vi "START SALES.vi"(11 "REFERENCES":T1) -> ()   [LabVIEW 2019]
uses:
  Controls/References Cluster.ctl
  Controls/Custom Calendar/Custom Calendar.xctl
  <vilib>/Utility/miscctls.llb/LVRowAndColumnTypeDef.ctl
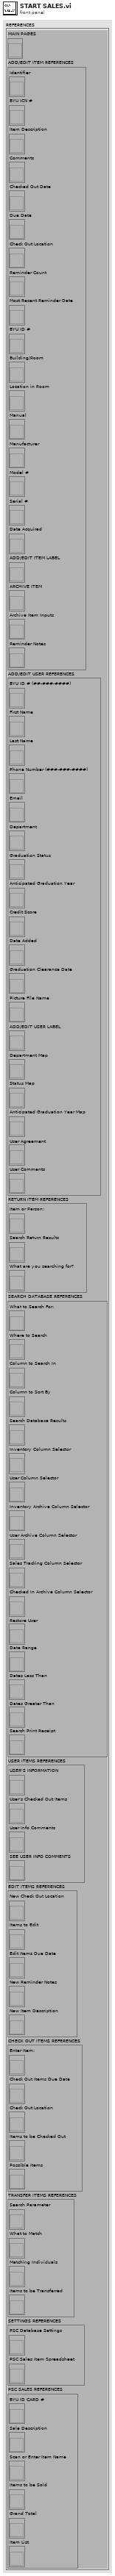
[diagram p1: front panel]
types:
  T1 = typedef "References Cluster.ctl" = cluster{"MAIN PAGES":refnum<vi>, "ADD/EDIT ITEM REFERENCES":cluster{"Identifier":refnum<vi>, "BYU ICN #":refnum<vi>, "Item Description":refnum<vi>, "Comments":refnum<vi>, "Checked Out Date":refnum<vi>, "Due Date":refnum<vi>, "Check Out Location":refnum<vi>, "Reminder Count":refnum<vi>, "Most Recent Reminder Date":refnum<vi>, "BYU ID #":refnum<vi>, "Building/Room":refnum<vi>, "Location in Room":refnum<vi>, "Manual":refnum<vi>, "Manufacturer":refnum<vi>, "Model #":refnum<vi>, "Serial #":refnum<vi>, "Date Acquired":refnum<vi>, "ADD/EDIT ITEM LABEL":refnum<vi>, "ARCHIVE ITEM":refnum<vi>, "Archive Item Inputs":refnum<vi>, "Reminder Notes":refnum<vi>}, "ADD/EDIT USER REFERENCES":cluster{"BYU ID # (##-###-####)":refnum<vi>, "First Name":refnum<vi>, "Last Name":refnum<vi>, "Phone Number (###-###-####)":refnum<vi>, "Email":refnum<vi>, "Department":refnum<vi>, "Graduation Status":refnum<vi>, "Anticipated Graduation Year":refnum<vi>, "Credit Score":refnum<vi>, "Date Added":refnum<vi>, "Graduation Clearance Date":refnum<vi>, "Picture File Name":refnum<vi>, "ADD/EDIT USER LABEL":refnum<vi>, "Department Map":refnum<vi>, "Status Map":refnum<vi>, "Anticipated Graduation Year Map":refnum<vi>, "User Agreement":refnum<vi>, "User Comments":refnum<vi>}, "RETURN ITEM REFERENCES":cluster{"Item or Person:":refnum<vi>, "Search Return Results":refnum<vi>, "What are you searching for?":refnum<vi>}, "SEARCH DATABASE REFERENCES":cluster{"What to Search For:":refnum<vi>, "Where to Search":refnum<vi>, "Column to Search In":refnum<vi>, "Column to Sort By":refnum<vi>, "Search Database Results":refnum<vi>, "Inventory Column Selector":refnum<vi>, "User Column Selector":refnum<vi>, "Inventory Archive Column Selector":refnum<vi>, "User Archive Column Selector":refnum<vi>, "Sales Tracking Column Selector":refnum<vi>, "Checked In Archive Column Selector":refnum<vi>, "Restore User":refnum<vi>, "Date Range":refnum<vi>, "Dates Less Than":refnum<vi>, "Dates Greater Than":refnum<vi>, "Search Print Receipt":refnum<vi>}, "USER ITEMS REFERENCES":cluster{"USER'S INFORMATION":refnum<vi>, "User's Checked Out Items":refnum<vi>, "User Info Comments":refnum<vi>, "SEE USER INFO COMMENTS":refnum<vi>}, "EDIT ITEMS REFERENCES":cluster{"New Check Out Location":refnum<vi>, "Items to Edit":refnum<vi>, "Edit Items Due Date":refnum<vi>, "New Reminder Notes":refnum<vi>, "New Item Description":refnum<vi>}, "CHECK OUT ITEMS REFERENCES":cluster{"Enter Item:":refnum<vi>, "Check Out Items Due Date":refnum<vi>, "Check Out Location":refnum<vi>, "Items to be Checked Out":refnum<vi>, "Possible Items":refnum<vi>}, "TRANSFER ITEMS REFERENCES":cluster{"Search Parameter":refnum<vi>, "What to Match":refnum<vi>, "Matching Individuals":refnum<vi>, "Items to be Transferred":refnum<vi>}, "SETTINGS REFERENCES":cluster{"PSC Database Settings":refnum<vi>, "PSC Sales Item Spreadsheet":refnum<vi>}, "PSC SALES REFERENCES":cluster{"BYU ID CARD #":refnum<vi>, "Sale Description":refnum<vi>, "Scan or Enter Item Name":refnum<vi>, "Items to be Sold":refnum<vi>, "Grand Total":refnum<vi>, "Item List":refnum<vi>}}
  T2 = typedef "LVRowAndColumnTypeDef.ctl" = cluster{"Row":i32, "Column":i32}
  T3 = cluster{"BYU ID CARD #":refnum<vi>, "Sale Description":refnum<vi>, "Scan or Enter Item Name":refnum<vi>, "Items to be Sold":refnum<vi>, "Grand Total":refnum<vi>, "Item List":refnum<vi>}
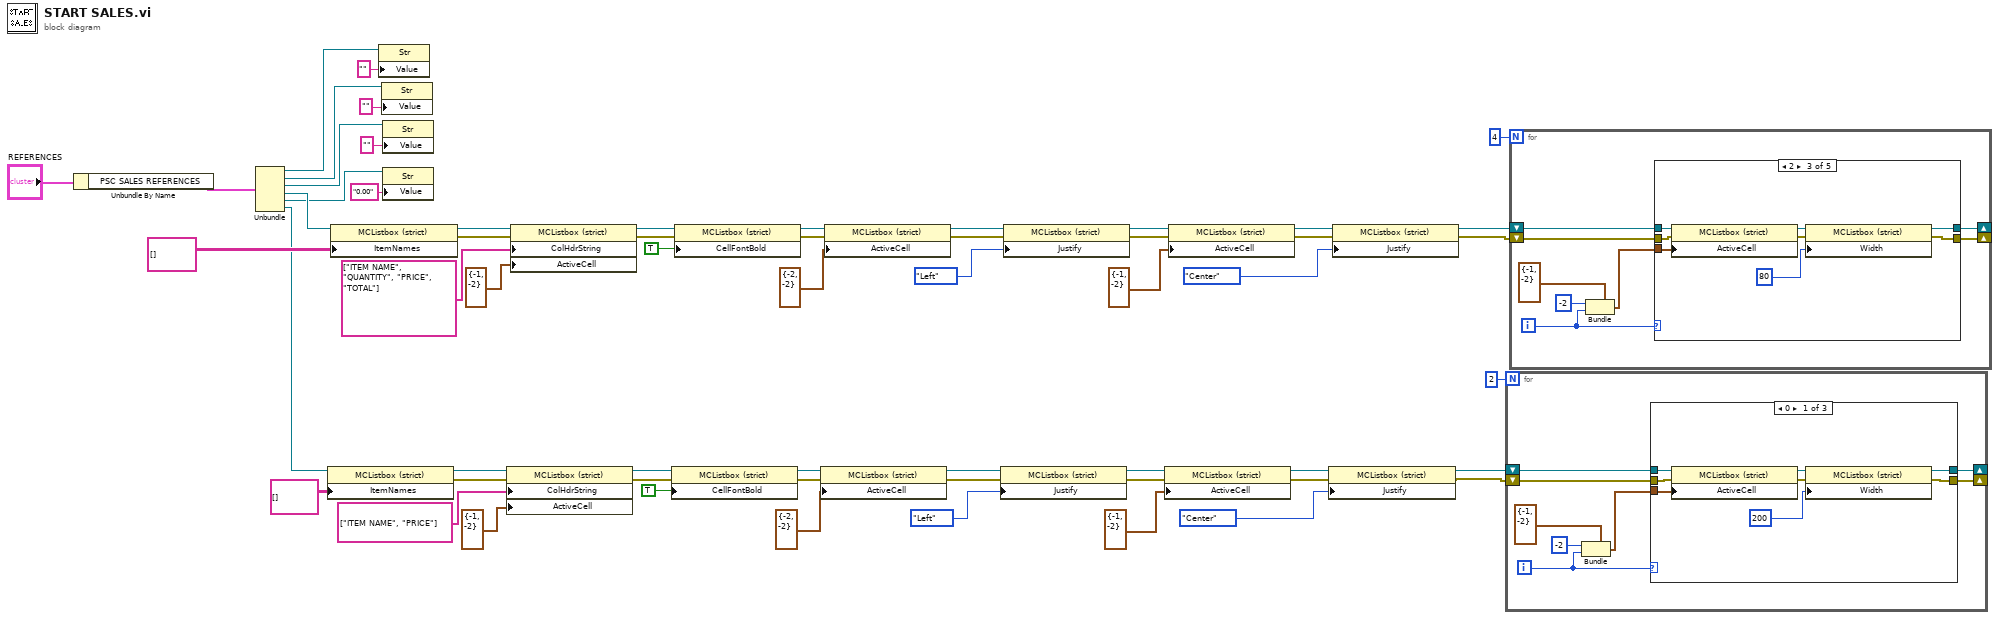
[diagram p0: block diagram]
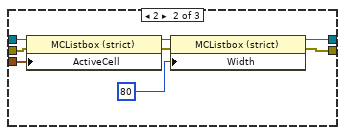
[diagram p2: hidden frame]
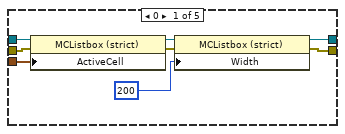
[diagram p4: hidden frame]
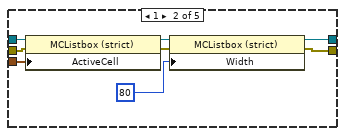
[diagram p5: hidden frame]
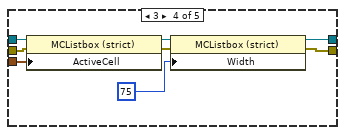
[diagram p6: hidden frame]
diagram:
  n1 = Unbundle By Name("REFERENCES") -> ("PSC SALES REFERENCES"=w57:T3)
  n2 = Unbundle(w57) -> ("BYU ID CARD #"=w32:refnum<vi>, "Sale Description"=w29:refnum<vi>, "Scan or Enter Item Name"=w27:refnum<vi>, "Items to be Sold"=w38:refnum<vi>, "Grand Total"=w25:refnum<vi>, "Item List"=w1:refnum<vi>)
  n3 = property class="MCListbox (strict)"(reference=w1, "ItemNames"=string[][] [] ("Item Names")) -> (reference out=w8:refnum<vi>, error out=w7:errorcluster)  [unwired: 1 in]
  n4 = property class="MCListbox (strict)"(reference=w38, "ItemNames"=string[][] [] ("Item Names")) -> (reference out=w40:refnum<vi>, error out=w39:errorcluster)  [unwired: 1 in]
  n5 = property class="Str"(reference=w32, "Value"="") -> ()  [unwired: 1 in, 2 out]
  n6 = property class="Str"(reference=w29, "Value"="") -> ()  [unwired: 1 in, 2 out]
  n7 = property class="Str"(reference=w27, "Value"="") -> ()  [unwired: 1 in, 2 out]
  n8 = property class="Str"(reference=w25, "Value"="0.00") -> ()  [unwired: 1 in, 2 out]
  n9 = property class="MCListbox (strict)"(reference=w8, error in=w7, "ColHdrString"=string[] ["ITEM NAME", "PRICE"] ("Column Header Strings[]"), "ActiveCell"=T2 {"Row"=-1, "Column"=-2} ("Active Cell:Active Cell")) -> (reference out=w23:refnum<vi>, error out=w22:errorcluster)
  n10 = property class="MCListbox (strict)"(reference=w40, error in=w39, "ColHdrString"=string[] ["ITEM NAME", "QUANTITY", "PRICE", "TOTAL"] ("Column Header Strings[]"), "ActiveCell"=T2 {"Row"=-1, "Column"=-2} ("Active Cell:Active Cell")) -> (reference out=w55:refnum<vi>, error out=w54:errorcluster)
  n11 = property class="MCListbox (strict)"(reference=w23, error in=w22, "CellFontBold"=TRUE ("Active Cell:Cell Font:Bold")) -> (reference out=w20:refnum<vi>, error out=w19:errorcluster)
  n12 = property class="MCListbox (strict)"(reference=w55, error in=w54, "CellFontBold"=TRUE ("Active Cell:Cell Font:Bold")) -> (reference out=w52:refnum<vi>, error out=w51:errorcluster)
  n13 = property class="MCListbox (strict)"(reference=w20, error in=w19, "ActiveCell"=T2 {"Row"=-2, "Column"=-2} ("Active Cell:Active Cell")) -> (reference out=w17:refnum<vi>, error out=w16:errorcluster)
  n14 = property class="MCListbox (strict)"(reference=w52, error in=w51, "ActiveCell"=T2 {"Row"=-2, "Column"=-2} ("Active Cell:Active Cell")) -> (reference out=w49:refnum<vi>, error out=w48:errorcluster)
  n15 = property class="MCListbox (strict)"(reference=w17, error in=w16, "Justify"=enum16{"Left", "Center", "Right"}."Left" ("Active Cell:Cell Justification")) -> (reference out=w12:refnum<vi>, error out=w11:errorcluster)
  n16 = property class="MCListbox (strict)"(reference=w49, error in=w48, "Justify"=enum16{"Left", "Center", "Right"}."Left" ("Active Cell:Cell Justification")) -> (reference out=w44:refnum<vi>, error out=w43:errorcluster)
  n17 = property class="MCListbox (strict)"(reference=w12, error in=w11, "ActiveCell"=T2 {"Row"=-1, "Column"=-2} ("Active Cell:Active Cell")) -> (reference out=w13:refnum<vi>, error out=w14:errorcluster)
  n18 = property class="MCListbox (strict)"(reference=w44, error in=w43, "ActiveCell"=T2 {"Row"=-1, "Column"=-2} ("Active Cell:Active Cell")) -> (reference out=w45:refnum<vi>, error out=w46:errorcluster)
  n19 = property class="MCListbox (strict)"(reference=w13, error in=w14, "Justify"=enum16{"Left", "Center", "Right"}."Center" ("Active Cell:Cell Justification")) -> (reference out=w3:refnum<vi>, error out=w2:errorcluster)
  n20 = property class="MCListbox (strict)"(reference=w45, error in=w46, "Justify"=enum16{"Left", "Center", "Right"}."Center" ("Active Cell:Cell Justification")) -> (reference out=w34:refnum<vi>, error out=w33:errorcluster)
  n21 = for {
    N: 2 -> [_]
    shift-right: [w61] -> _
    shift-left: w3 -> [w63]
    shift-right: [w60] -> _
    shift-left: w2 -> [w62]
    i -> [w65]
    n22 = Bundle(cluster=T2 {"Row"=-1, "Column"=-2} ("Active Cell:Active Cell"), "Row"=-2, "Column"=w65) -> (w64:T2)
    n23 = case shown="0" w65 {
      tunnel: w64 -> [w74 w75 _]
      tunnel: w63 -> [w73 w80 w84]
      tunnel: w62 -> [w72 w79 w83]
      tunnel: [w68 w77 w84] -> w61
      tunnel: [w67 w76 w83] -> w60
      frame 0 {
        n24 = property class="MCListbox (strict)"(reference=w73, error in=w72, "ActiveCell"=w74) -> (reference out=w71:refnum<vi>, error out=w70:errorcluster)
        n25 = property class="MCListbox (strict)"(reference=w71, error in=w70, "Width"=u32 200 ("Active Cell:Cell Size:Width")) -> (reference out=w68:refnum<vi>, error out=w67:errorcluster)
      }
      frame 2 {
        n26 = property class="MCListbox (strict)"(reference=w80, error in=w79, "ActiveCell"=w75) -> (reference out=w78:refnum<vi>, error out=w82:errorcluster)
        n27 = property class="MCListbox (strict)"(reference=w78, error in=w82, "Width"=u32 80 ("Active Cell:Cell Size:Width")) -> (reference out=w77:refnum<vi>, error out=w76:errorcluster)
      }
      frame Default {
      }
    }
  }
  n28 = for {
    N: 4 -> [_]
    shift-right: [w87] -> _
    shift-left: w34 -> [w89]
    shift-right: [w86] -> _
    shift-left: w33 -> [w88]
    i -> [w91]
    n29 = Bundle(cluster=T2 {"Row"=-1, "Column"=-2} ("Active Cell:Active Cell"), "Row"=-2, "Column"=w91) -> (w90:T2)
    n30 = case shown="2" w91 {
      tunnel: w90 -> [w100 w101 w109 w117 _]
      tunnel: w89 -> [w99 w105 w114 w122 w126]
      tunnel: w88 -> [w98 w104 w113 w121 w125]
      tunnel: [w94 w103 w111 w119 w126] -> w87
      tunnel: [w93 w102 w110 w118 w125] -> w86
      frame 0 {
        n31 = property class="MCListbox (strict)"(reference=w99, error in=w98, "ActiveCell"=w100) -> (reference out=w97:refnum<vi>, error out=w96:errorcluster)
        n32 = property class="MCListbox (strict)"(reference=w97, error in=w96, "Width"=u32 200 ("Active Cell:Cell Size:Width")) -> (reference out=w94:refnum<vi>, error out=w93:errorcluster)
      }
      frame 1 {
        n33 = property class="MCListbox (strict)"(reference=w105, error in=w104, "ActiveCell"=w101) -> (reference out=w108:refnum<vi>, error out=w107:errorcluster)
        n34 = property class="MCListbox (strict)"(reference=w108, error in=w107, "Width"=u32 80 ("Active Cell:Cell Size:Width")) -> (reference out=w103:refnum<vi>, error out=w102:errorcluster)
      }
      frame 2 {
        n35 = property class="MCListbox (strict)"(reference=w114, error in=w113, "ActiveCell"=w109) -> (reference out=w112:refnum<vi>, error out=w116:errorcluster)
        n36 = property class="MCListbox (strict)"(reference=w112, error in=w116, "Width"=u32 80 ("Active Cell:Cell Size:Width")) -> (reference out=w111:refnum<vi>, error out=w110:errorcluster)
      }
      frame 3 {
        n37 = property class="MCListbox (strict)"(reference=w122, error in=w121, "ActiveCell"=w117) -> (reference out=w120:refnum<vi>, error out=w124:errorcluster)
        n38 = property class="MCListbox (strict)"(reference=w120, error in=w124, "Width"=u32 75 ("Active Cell:Cell Size:Width")) -> (reference out=w119:refnum<vi>, error out=w118:errorcluster)
      }
      frame Default {
      }
    }
  }
